vi "Event Handle Loop_Draw_Button.vi"(7 "Active":bool, 8 "error in (no error)":errorcluster, 10 "Picture In":picture, 11 "QMenu Class in":refnum<class "QMenu Class.lvclass">) -> (0 "error out":errorcluster, 2 "Picture Out":picture, 3 "QMenu Class out":refnum<class "QMenu Class.lvclass">)   [LabVIEW 2020, in "QTab.lvlib" / "QMenu Class.lvclass"]
uses:
  QMenu Class.lvclass
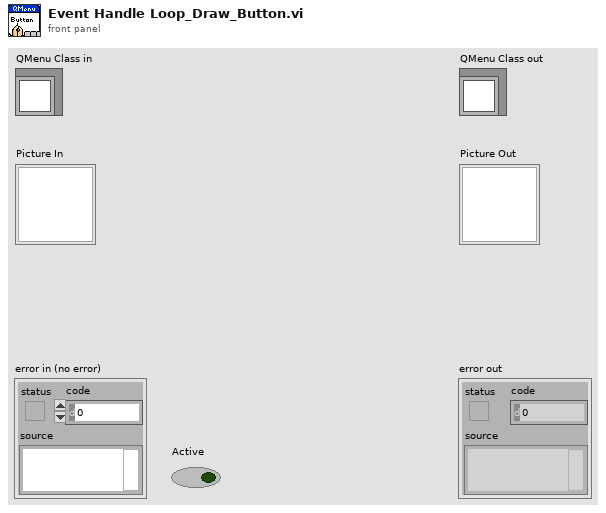
[diagram p1: front panel]
types:
  T1 = typedef "imagedata.ctl" = cluster{"image type":i32, "image depth":i32, "image":u8[], "mask":u8[], "colors":u32[], "Rectangle":cluster{"left":i16, "top":i16, "right":i16, "bottom":i16}}
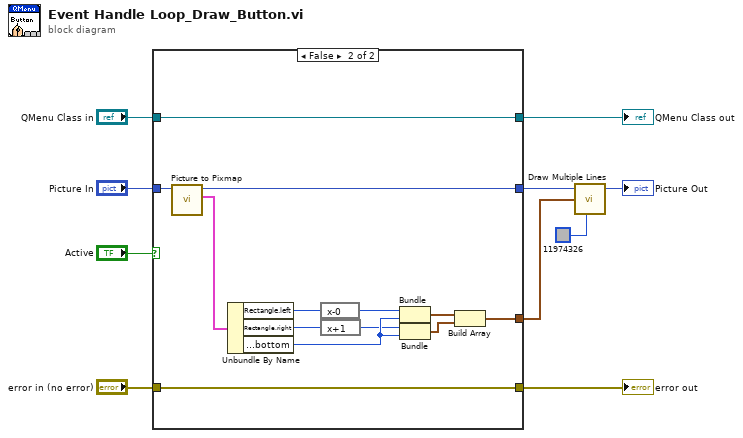
[diagram p0: block diagram]
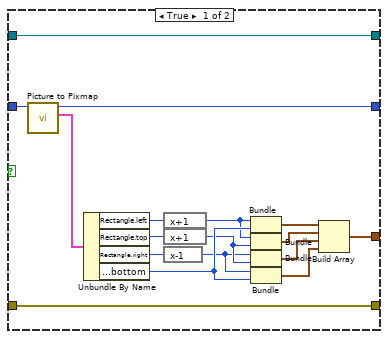
[diagram p2: hidden frame]
diagram:
  n1 = case shown="False" "Active" {
    tunnel: "Picture In" -> [w27 w32]
    tunnel: [w13 w28] -> w4
    tunnel: "QMenu Class in" -> [w11 w39]
    tunnel: [w11 w39] -> w7
    tunnel: "error in (no error)" -> [w14 w38]
    tunnel: [w14 w38] -> w5
    tunnel: [w12 w36] -> w3
    frame True {
      n2 = call <vilib>:"Picture to Pixmap.vi"("picture"=w27) -> ("image data"=w26:T1, "new picture"=w13:picture)  [unwired: 9 in]
      n3 = Unbundle By Name(w26) -> ("Rectangle.left"=w18:i16, "Rectangle.top"=w20:i16, "Rectangle.right"=w16:i16, "Rectangle.bottom"=w25:i16)
      n4 = expression code="x+1"(w18) -> (w17:i16)
      n5 = expression code="x+1"(w20) -> (w19:i16)
      n6 = expression code="x-1"(w16) -> (w15:i16)
      n7 = Bundle("left"=w17, "bottom"=w25) -> (w24:cluster{"left":i16, "bottom":i16})  [unwired: 1 in]
      n8 = Bundle("left"=w17, "top"=w19) -> (w23:cluster{"left":i16, "top":i16})  [unwired: 1 in]
      n9 = Bundle("right"=w15, "top"=w19) -> (w22:cluster{"right":i16, "top":i16})  [unwired: 1 in]
      n10 = Bundle("right"=w15, "bottom"=w25) -> (w21:cluster{"right":i16, "bottom":i16})  [unwired: 1 in]
      n11 = Build Array(w24, w23, w22, w21) -> (w12:cluster{"right":i16, "bottom":i16}[])
    }
    frame False {
      n12 = call <vilib>:"Picture to Pixmap.vi"("picture"=w32) -> ("image data"=w35:T1, "new picture"=w28:picture)  [unwired: 9 in]
      n13 = Unbundle By Name(w35) -> ("Rectangle.left"=w31:i16, "Rectangle.right"=w30:i16, "Rectangle.bottom"=w33:i16)
      n14 = expression code="x-0"(w31) -> (w34:i16)
      n15 = expression code="x+1"(w30) -> (w29:i16)
      n16 = Bundle("left"=w34, "bottom"=w33) -> (w40:cluster{"left":i16, "bottom":i16})  [unwired: 1 in]
      n17 = Bundle("right"=w29, "bottom"=w33) -> (w37:cluster{"right":i16, "bottom":i16})  [unwired: 1 in]
      n18 = Build Array(w40, w37) -> (w36:cluster{"right":i16, "bottom":i16}[])
    }
  }
  "error out" <- w5
  "QMenu Class out" <- w7
  n19 = call <vilib>:"Draw Multiple Lines.vi"("picture"=w4, "line endpoints"=w3, "color(black)"=u32 11974326) -> ("new picture"=→"Picture Out":picture)  [unwired: 6 in]
